vi "pmu_Build Class CFG-3.vi"(8 "error in (no error)":errorcluster, 11 "CFG-3":T1={"PMU ID"=1, "global PMU ID"=1, "time base"=10000000, "nominal frequency"=enum."60 Hz", "reporting rate"=60, "station name"="", "data format"=15, "phasor channels"=[], "analog channels"=[], "digital channels"=[]} {"data format" format="%016b"; "phasor channels"."phasor unit" items=["Voltage [V]"=0, "Current [A]"=16777216]; "phasor channels"."data modification flag" format="%016b"; "digital channels"."digital unit" format="%08x"}) -> (0 "error out":errorcluster, 3 "CFG-3 class":T5={"station name"="", "PMU ID"=1, "global PMU ID"=1, "time base"=1, "nominal frequency"=enum."60 Hz", "reporting rate"=0, "phasor number"=0, "analog number"=0, "digital number"=0, "channel names"=[], "phasor scale first 4 bytes"=[], "phasor scale factors"=[], "phasor angle offsets [rad]"=[], "analog scale factors"=[], "analog magnitude offsets"=[], "digital units"=[], "data format"=15, "number of PMUs"=1} {"digital units" format="%.0x"})   [LabVIEW 2013, in "NI_EP_PMU.lvlib"]
uses:
  <vilib>/addons/Electrical Power/PMU/NI_EP_PMU.lvlib
  <vilib>/addons/Electrical Power/PMU/Common/Controls/pmu_CFG-3 Class.ctl
  <vilib>/addons/Electrical Power/PMU/Common/Controls/pmu_CFG-3 Input.ctl
  <vilib>/addons/Electrical Power/PMU/Common/Controls/pmu_CFG-3 Phasor Channels.ctl
  <vilib>/addons/Electrical Power/PMU/Common/Controls/pmu_CFG-3 Analog Channels.ctl
  <vilib>/addons/Electrical Power/PMU/Common/Controls/pmu_Digital Channel.ctl
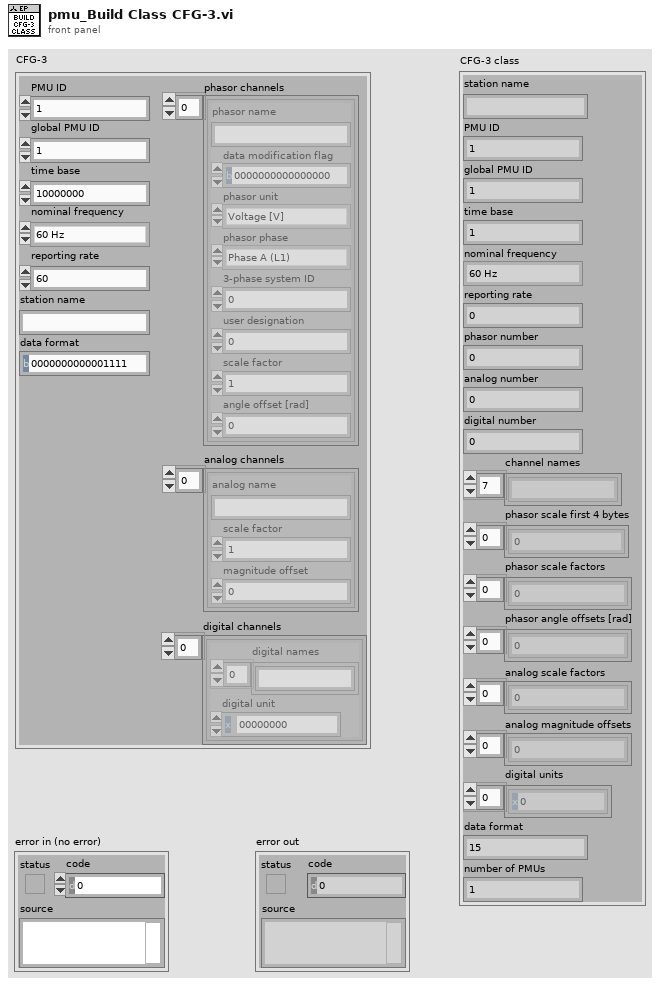
[diagram p1: front panel]
types:
  T1 = typedef "NI_EP_PMU.lvlib/pmu_CFG-3 Input.ctl" = cluster{"PMU ID":u16, "global PMU ID":u64, "time base":u32, "nominal frequency":enum16{"50 Hz", "60 Hz"}, "reporting rate":i16, "station name":string, "data format":u16, "phasor channels":T2[], "analog channels":T3[], "digital channels":T4[]}
  T2 = typedef "NI_EP_PMU.lvlib/pmu_CFG-3 Phasor Channels.ctl" = cluster{"phasor name":string, "data modification flag":u16, "phasor unit":u32, "phasor phase":enum16{"Phase A (L1)", "Phase B (L2)", "Phase C (L3)", "Phase N", "Positive sequence", "Negative sequence", "Zero sequence"}, "3-phase system ID":u8, "user designation":u8, "scale factor":sgl, "angle offset [rad]":sgl}
  T3 = typedef "NI_EP_PMU.lvlib/pmu_CFG-3 Analog Channels.ctl" = cluster{"analog name":string, "scale factor":sgl, "magnitude offset":sgl}
  T4 = typedef "NI_EP_PMU.lvlib/pmu_Digital Channel.ctl" = cluster{"digital names":string[], "digital unit":u32}
  T5 = typedef "NI_EP_PMU.lvlib/pmu_CFG-3 Class.ctl" = cluster{"station name":string, "PMU ID":u16, "global PMU ID":u64, "time base":u32, "nominal frequency":enum16{"50 Hz", "60 Hz"}, "reporting rate":i16, "phasor number":u16, "analog number":u16, "digital number":u16, "channel names":string[], "phasor scale first 4 bytes":u32[], "phasor scale factors":sgl[], "phasor angle offsets [rad]":sgl[], "analog scale factors":sgl[], "analog magnitude offsets":sgl[], "digital units":u32[], "data format":u16, "number of PMUs":u16}
  T6 = enum16{"Phase A (L1)", "Phase B (L2)", "Phase C (L3)", "Phase N", "Positive sequence", "Negative sequence", "Zero sequence"}
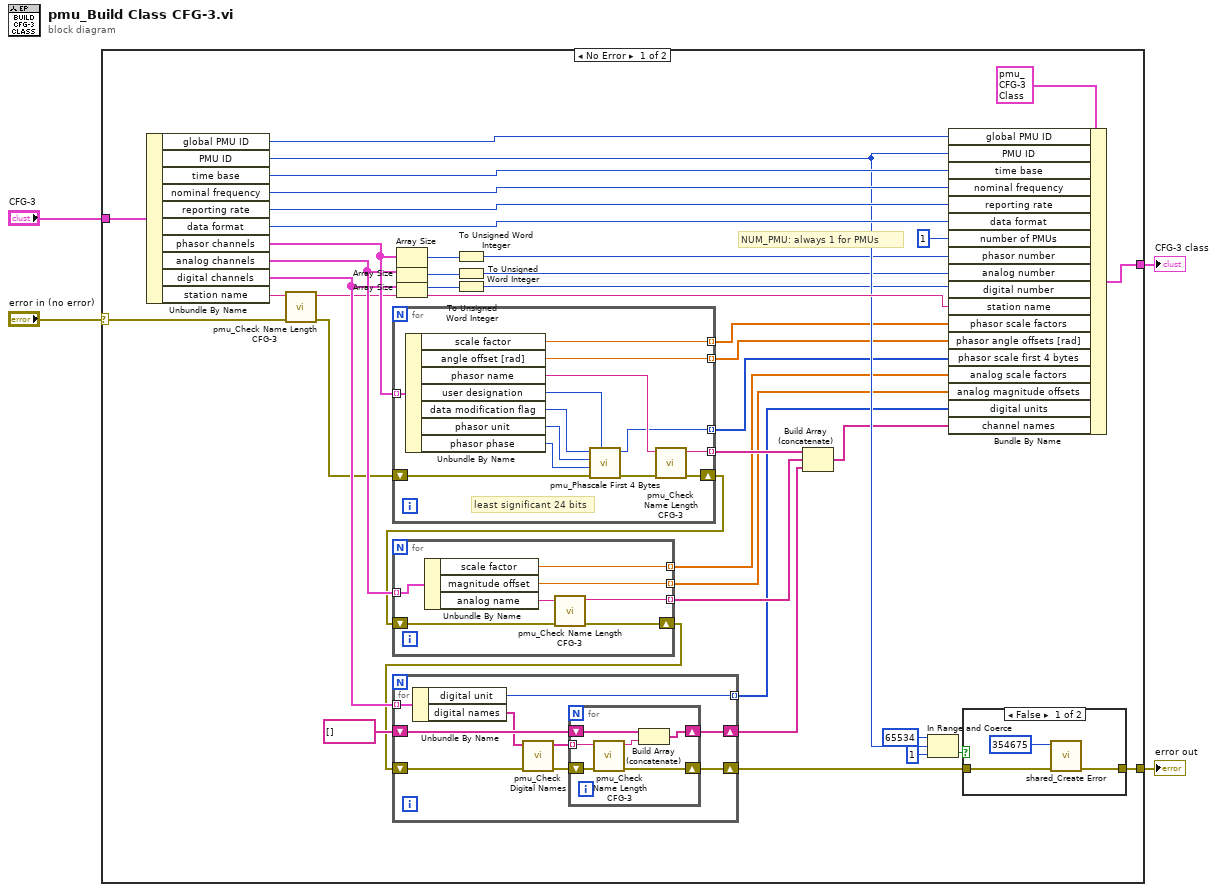
[diagram p0: block diagram]
diagram:
  n1 = case shown="No Error" "error in (no error)" {
    selector: "error in (no error)" -> [w31 w85]
    tunnel: "CFG-3" -> [w45 _]
    tunnel: [w26 w85] -> w2
    tunnel: [w17 _] -> w1
    frame No Error {
      # "NUM_PMU: always 1 for PMUs"
      n2 = Unbundle By Name(w45) -> ("global PMU ID"=w16:u64, "PMU ID"=w28:u16, "time base"=w44:u32, "nominal frequency"=w43:enum16{"50 Hz", "60 Hz"}, "reporting rate"=w42:i16, "data format"=w41:u16, "phasor channels"=w38:T2[], "analog channels"=w37:T3[], "digital channels"=w36:T4[], "station name"=w35:string)
      n3 = call <vilib>:"pmu_Check Name Length CFG-3.vi"("error in (no error)"=w31, "name in"=w35) -> ("error out"=w15:errorcluster, "name out"=w34:string)  [unwired: 8 in]
      n4 = for {
        tunnel: w38 -> [w84] mode=indexing
        shift-right: [w83] -> w11
        shift-left: w15 -> [w81]
        tunnel: [w82] -> w33 mode=indexing
        tunnel: [w74] -> w13 mode=indexing
        tunnel: [w73] -> w14 mode=indexing
        tunnel: [w72] -> w12 mode=indexing
        # "least significant 24 bits"
        n5 = Unbundle By Name(w84) -> ("scale factor"=w73:sgl, "angle offset [rad]"=w74:sgl, "phasor name"=w75:string, "user designation"=w76:u8, "data modification flag"=w77:u16, "phasor unit"=w78:u32, "phasor phase"=w79:T6)
        n6 = call <vilib>:"pmu_Phascale First 4 Bytes.vi"("user designation"=w76, "error in (no error)"=w81, "phasor phase"=w79, "phasor unit"=w78, "data modification flag"=w77) -> ("error out"=w80:errorcluster, "PHSCALE first 4 bytes"=w72:u32)  [unwired: 5 in]
        n7 = call <vilib>:"pmu_Check Name Length CFG-3.vi"("error in (no error)"=w80, "name in"=w75) -> ("error out"=w83:errorcluster, "name out"=w82:string)  [unwired: 8 in]
      }
      n8 = for {
        tunnel: w37 -> [w71] mode=indexing
        shift-right: [w70] -> w10
        shift-left: w11 -> [w69]
        tunnel: [w68] -> w32 mode=indexing
        tunnel: [w67] -> w9 mode=indexing
        tunnel: [w66] -> w8 mode=indexing
        n9 = Unbundle By Name(w71) -> ("scale factor"=w67:sgl, "magnitude offset"=w66:sgl, "analog name"=w65:string)
        n10 = call <vilib>:"pmu_Check Name Length CFG-3.vi"("error in (no error)"=w69, "name in"=w65) -> ("error out"=w70:errorcluster, "name out"=w68:string)  [unwired: 8 in]
      }
      n11 = for {
        tunnel: w36 -> [w58] mode=indexing
        tunnel: [w57] -> w7 mode=indexing
        shift-right: [w54] -> w39
        shift-left: string[] [] ("element") -> [w55]
        shift-right: [w56] -> w5
        shift-left: w10 -> [w50]
        n12 = Unbundle By Name(w58) -> ("digital unit"=w57:u32, "digital names"=w53:string[])
        n13 = call <vilib>:"pmu_Check Digital Names.vi"("error in (no error)"=w50, "digital names in"=w53) -> ("error out"=w51:errorcluster, "digital names out"=w52:string[])  [unwired: 8 in]
        n14 = for {
          tunnel: w52 -> [w64] mode=indexing
          shift-right: [w62] -> w56
          shift-left: w51 -> [w63]
          shift-right: [w59] -> w54
          shift-left: w55 -> [w60]
          n15 = call <vilib>:"pmu_Check Name Length CFG-3.vi"("error in (no error)"=w63, "name in"=w64) -> ("error out"=w62:errorcluster, "name out"=w61:string)  [unwired: 8 in]
          n16 = Build Array (concatenate)(w60, w61) -> (w59:string[])
        }
      }
      n17 = Array Size(array=w38) -> (size(s)=w24:i32)
      n18 = Array Size(array=w37) -> (size(s)=w22:i32)
      n19 = Array Size(array=w36) -> (size(s)=w20:i32)
      n20 = To Unsigned Word Integer(number=w24) -> (unsigned 16bit integer=w23:u16)
      n21 = To Unsigned Word Integer(number=w22) -> (unsigned 16bit integer=w21:u16)
      n22 = To Unsigned Word Integer(number=w20) -> (unsigned 16bit integer=w19:u16)
      n23 = Build Array (concatenate)(w33, w32, w39) -> (w6:string[])
      n24 = In Range and Coerce(upper limit=u16 65534, x=w28, lower limit=u16 1) -> (In Range?=w27:bool)  [unwired: 1 out]
      n25 = Bundle By Name(cluster=T5 {"station name"="", "PMU ID"=0, "global PMU ID"=38528, "time base"=1, "nominal frequency"=enum."60 Hz", "reporting rate"=0, "phasor number"=0, "analog number"=0, "digital number"=0, "channel names"=[], "phasor scale first 4 bytes"=[], "phasor scale factors"=[], "phasor angle offsets [rad]"=[], "analog scale factors"=[], "analog magnitude offsets"=[], "digital units"=[], "data format"=0, "number of PMUs"=0} ("CFG-3 class"), "global PMU ID"=w16, "PMU ID"=w28, "time base"=w44, "nominal frequency"=w43, "reporting rate"=w42, "data format"=w41, "number of PMUs"=u16 1, "phasor number"=w23, "analog number"=w21, "digital number"=w19, "station name"=w34, "phasor scale factors"=w14, "phasor angle offsets [rad]"=w13, "phasor scale first 4 bytes"=w12, "analog scale factors"=w9, "analog magnitude offsets"=w8, "digital units"=w7, "channel names"=w6) -> (w17:T5)
      n26 = case shown="False" w27 {
        tunnel: [w47 w49] -> w26
        tunnel: w5 -> [w46 w49]
        frame False {
          n27 = call <vilib>:"shared_Create Error.vi"("error in (no error)"=w46, "error code (0)"=354675 ("code")) -> ("error out"=w47:errorcluster)  [unwired: 9 in]
        }
        frame True {
        }
      }
    }
    frame Error {
    }
  }
  "CFG-3 class" <- w1
  "error out" <- w2
